vi "习题3.1.vi"() -> ()   [LabVIEW 2017]
panel:
  out "cos(x)":dbl
  out "sin(x)":dbl
  in  "数值":dbl
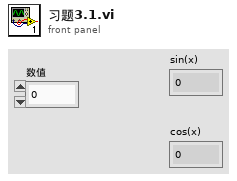
[diagram p1: front panel]
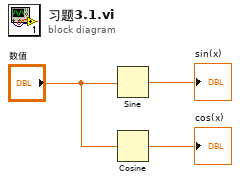
[diagram p0: block diagram]
diagram:
  n1 = Sine(x="数值") -> (sin(x)=→"sin(x)":dbl)
  n2 = Cosine(x="数值") -> (cos(x)=→"cos(x)":dbl)
